vi "Decorate Root.vi"(10 "Stop When Parent Stopped":bool=TRUE) -> (5 "Actor out":refnum<class "Actor.lvclass">)   [LabVIEW 2025, in "jettl.lvlib" / "Core Actor.lvlib"]
uses:
  Core Actor.lvlib
  Actor/Actor.lvclass
  Core Actor/Core Actor.lvclass
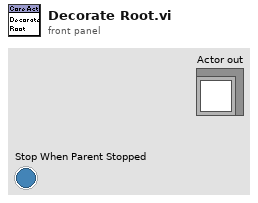
[diagram p1: front panel]
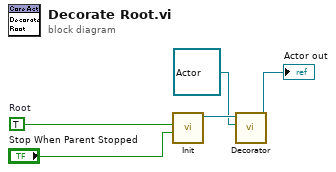
[diagram p0: block diagram]
diagram:
  w2 = TRUE  # Root
  n1 = call "Init.vi"("Stop When Parent Stopped"="Stop When Parent Stopped", "Root"=w2) -> ("Core Actor out"=w4:refnum<class "Core Actor.lvclass">)  [unwired: 9 in]
  n2 = call-dynamic "Decorator.vi"("Actor"=refnum<class "Actor.lvclass"> refnum, "Core Actor in"=w4) -> ("Core Actor out"=→"Actor out":refnum<class "Core Actor.lvclass">)  [unwired: 9 in]
